vi "testSendEvtToClient.vi"(8 "error in (no error)":errorcluster) -> (0 "error out":errorcluster)   [LabVIEW 2018]
doc: "This VI generates 50 events and sends them from TCP server to TCP client."
uses:
  <vilib>/addons/_JKI Toolkits/Caraya/classes/Assert/Assert Equal Value_Variant.vi
  src/TcpServer/TcpServer.lvclass
  <vilib>/addons/_JKI Toolkits/Caraya/classes/Test/Test.lvclass
  <vilib>/addons/_JKI Toolkits/Caraya/classes/Assert/Assert.lvclass
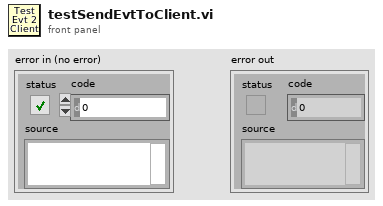
[diagram p1: front panel]
types:
  T1 = cluster{"CmdRead":refnum<user-event>, "EvtRead":refnum<user-event>, "GenRead":refnum<user-event>}
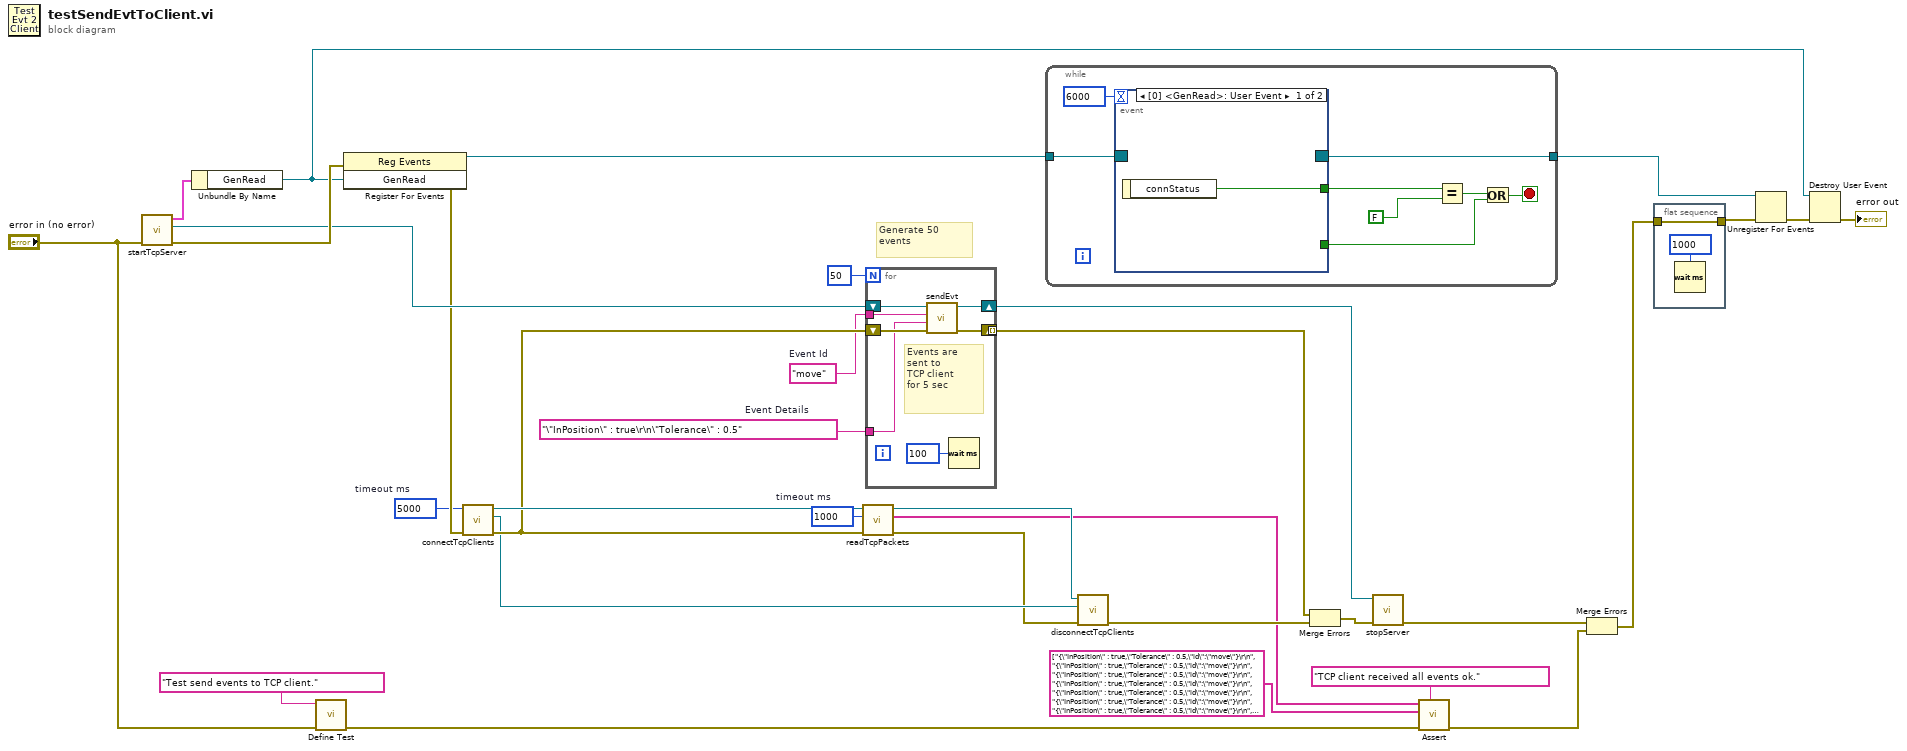
[diagram p0: block diagram]
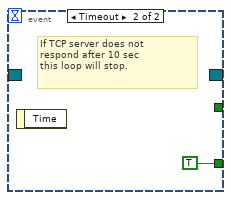
[diagram p2: hidden frame]
diagram:
  w3 = 1000  # timeout ms
  w4 = 5000  # timeout ms
  w9 = "\"InPosition\" : true\r\n\"Tolerance\" : 0.5"  # Event Details
  w8 = "move"  # Event Id
  # "Generate 50 \nevents"
  n1 = call "startTcpServer.vi"("error in (no error)"="error in (no error)") -> ("error out"=w21:errorcluster, "TcpServer out"=w18:refnum<class "TcpServer.lvclass">, "UserEvents"=w28:T1)  [unwired: 8 in]
  n2 = Unbundle By Name(w28) -> ("GenRead"=w1:refnum<user-event>)
  n3 = call <vilib>:"Define Test.vi"("error in (no error)"="error in (no error)", "Label (VI Title)"="Test send events to TCP client.") -> ("error out"=w15:errorcluster)  [unwired: 9 in]
  n4 = register-events(error in=w21, w1) -> (reference out=w33:refnum<event-registration>, error out=w10:errorcluster)  [unwired: 1 in]
  n5 = call "connectTcpClients.vi"("error in (no error)"=w10, "timeout ms"=w4) -> ("error out"=w26:errorcluster, "tel connection ID out"=w24:refnum<k5>, "cmd connection ID out"=w27:refnum<k5>)  [unwired: 7 in]
  n6 = call "readTcpPackets.vi"("error in (no error)"=w26, "timeout ms"=w3, "connection ID in"=w27) -> ("error out"=w23:errorcluster, "TCP packets"=w16:string[], "connection ID out"=w25:refnum<k5>)  [unwired: 6 in]
  n7 = for {
    N: 50 -> [_]
    tunnel: w9 -> [w35]
    tunnel: w8 -> [w40]
    shift-right: [w37] -> w11
    shift-left: w18 -> [w39]
    shift-right: [w34] -> w5
    shift-left: w26 -> [w38]
    tunnel: [w34] -> _ mode=indexing
    # "Events are\nsent to\nTCP client\nfor 5 sec"
    n8 = call "sendEvt.vi"("error in (no error)"=w38, "Event Details"=w35, "Event Id"=w40, "tcpServer in"=w39) -> ("error out"=w34:errorcluster, "tcpServer out"=w37:refnum<class "TcpServer.lvclass">)  [unwired: 6 in]
    n9 = Wait (ms)(milliseconds to wait=u32 100) -> ()  [unwired: 1 out]
  }
  n10 = while {
    tunnel: w33 -> [w48]
    tunnel: [w47] -> w32
    stop <- w42 stop-if-true
    n11 = event shown="[0] <GenRead>: User Event" {
      selector: w48 -> [_ _]
      dyn-events: [_ _] -> w47
      timeout: 6000 -> [_ _]
      tunnel: [w49 _] -> w46
      tunnel: [_ TRUE] -> w43
      event User Event {
        n12 = event-data() -> ("connStatus"=w49:bool)  [unwired: 1 in]
      }
      event Timeout {
        # "If TCP server does not\nrespond after 10 sec\nthis loop will stop."
        n13 = event-data() -> ()  [unwired: 1 in, 1 out]
      }
    }
    n14 = Equal?(x=w46, y=FALSE) -> (x = y?=w44:bool)
    n15 = Or(x=w44, y=w43) -> (x .or. y?=w42:bool)
  }
  n16 = call "disconnectTcpClients.vi"("error in (no error)"=w23, "tel connection ID in"=w24, "cmd connection ID in"=w25) -> ("error out"=w22:errorcluster)  [unwired: 8 in]
  n17 = Merge Errors(w5, w22) -> (w6:errorcluster)
  n18 = call "stopServer.vi"("error in (no error)"=w6, "tcpServer in"=w11) -> ("error out"=w30:errorcluster)  [unwired: 8 in, 1 out]
  n19 = call-poly <vilib>:"Assert.vi"("Label"="TCP client received all events ok.", "error in (no error)"=w15, "Y"=string[] ["{\"InPosition\" : true,\"Tolerance\" : 0.5,\"id\":\"move\"}\r\n", "{\"InPosition\" : true,\"Tolerance\" : 0.5,\"id\":\"move\"}\r\n", "{\"InPosition\" : true,\"Tolerance\" : 0.5,\"id\":\"move\"}\r\n", "{\"InPosition\" : true,\"Tolerance\" : 0.5,\"id\":\"move\"}\r\n", "{\"InPosition\" : true,\"Tolerance\" : 0.5,\"id\":\"move\"}\r\n", "{\"InPosition\" : true,\"Tolerance\" : 0.5,\"id\":\"move\"}\r\n", "{\"InPosition\" : true,\"Tolerance\" : 0.5,\"id\":\"move\"}\r\n", "{\"InPosition\" : true,\"Tolerance\" : 0.5,\"id\":\"move\"}\r\n", "{\"InPosition\" : true,\"Tolerance\" : 0.5,\"id\":\"move\"}\r\n", "{\"InPosition\" : true,\"Tolerance\" : 0.5,\"id\":\"move\"}\r\n", "{\"InPosition\" : true,\"Tolerance\" : 0.5,\"id\":\"move\"}\r\n", "{\"InPosition\" : true,\"Tolerance\" : 0.5,\"id\":\"move\"}\r\n", "{\"InPosition\" : true,\"Tolerance\" : 0.5,\"id\":\"move\"}\r\n", "{\"InPosition\" : true,\"Tolerance\" : 0.5,\"id\":\"move\"}\r\n", "{\"InPosition\" : true,\"Tolerance\" : 0.5,\"id\":\"move\"}\r\n", "{\"InPosition\" : true,\"Tolerance\" : 0.5,\"id\":\"move\"}\r\n", "{\"InPosition\" : true,\"Tolerance\" : 0.5,\"id\":\"move\"}\r\n", "{\"InPosition\" : true,\"Tolerance\" : 0.5,\"id\":\"move\"}\r\n", "{\"InPosition\" : true,\"Tolerance\" : 0.5,\"id\":\"move\"}\r\n", "{\"InPosition\" : true,\"Tolerance\" : 0.5,\"id\":\"move\"}\r\n", "{\"InPosition\" : true,\"Tolerance\" : 0.5,\"id\":\"move\"}\r\n", "{\"InPosition\" : true,\"Tolerance\" : 0.5,\"id\":\"move\"}\r\n", "{\"InPosition\" : true,\"Tolerance\" : 0.5,\"id\":\"move\"}\r\n", "{\"InPosition\" : true,\"Tolerance\" : 0.5,\"id\":\"move\"}\r\n", "{\"InPosition\" : true,\"Tolerance\" : 0.5,\"id\":\"move\"}\r\n", "{\"InPosition\" : true,\"Tolerance\" : 0.5,\"id\":\"move\"}\r\n", "{\"InPosition\" : true,\"Tolerance\" : 0.5,\"id\":\"move\"}\r\n", "{\"InPosition\" : true,\"Tolerance\" : 0.5,\"id\":\"move\"}\r\n", "{\"InPosition\" : true,\"Tolerance\" : 0.5,\"id\":\"move\"}\r\n", "{\"InPosition\" : true,\"Tolerance\" : 0.5,\"id\":\"move\"}\r\n", "{\"InPosition\" : true,\"Tolerance\" : 0.5,\"id\":\"move\"}\r\n", "{\"InPosition\" : true,\"Tolerance\" : 0.5,\"id\":\"move\"}\r\n", "{\"InPosition\" : true,\"Tolerance\" : 0.5,\"id\":\"move\"}\r\n", "{\"InPosition\" : true,\"Tolerance\" : 0.5,\"id\":\"move\"}\r\n", "{\"InPosition\" : true,\"Tolerance\" : 0.5,\"id\":\"move\"}\r\n", "{\"InPosition\" : true,\"Tolerance\" : 0.5,\"id\":\"move\"}\r\n", "{\"InPosition\" : true,\"Tolerance\" : 0.5,\"id\":\"move\"}\r\n", "{\"InPosition\" : true,\"Tolerance\" : 0.5,\"id\":\"move\"}\r\n", "{\"InPosition\" : true,\"Tolerance\" : 0.5,\"id\":\"move\"}\r\n", "{\"InPosition\" : true,\"Tolerance\" : 0.5,\"id\":\"move\"}\r\n", "{\"InPosition\" : true,\"Tolerance\" : 0.5,\"id\":\"move\"}\r\n", "{\"InPosition\" : true,\"Tolerance\" : 0.5,\"id\":\"move\"}\r\n", "{\"InPosition\" : true,\"Tolerance\" : 0.5,\"id\":\"move\"}\r\n", "{\"InPosition\" : true,\"Tolerance\" : 0.5,\"id\":\"move\"}\r\n", "{\"InPosition\" : true,\"Tolerance\" : 0.5,\"id\":\"move\"}\r\n", "{\"InPosition\" : true,\"Tolerance\" : 0.5,\"id\":\"move\"}\r\n", "{\"InPosition\" : true,\"Tolerance\" : 0.5,\"id\":\"move\"}\r\n", "{\"InPosition\" : true,\"Tolerance\" : 0.5,\"id\":\"move\"}\r\n", "{\"InPosition\" : true,\"Tolerance\" : 0.5,\"id\":\"move\"}\r\n", "{\"InPosition\" : true,\"Tolerance\" : 0.5,\"id\":\"move\"}\r\n"] ("array w/ subset deleted"), "X"=w16) -> ("error out"=w13:errorcluster)  [unwired: 7 in]
  n20 = Merge Errors(w30, w13) -> (w14:errorcluster)
  n21 = flat-sequence {
    tunnel: w14 -> [w51]
    tunnel: [w51] -> w29
    frame #0 {
      n22 = Wait (ms)(milliseconds to wait=u32 1000) -> ()  [unwired: 1 out]
    }
  }
  n23 = Unregister For Events(event registration refnum=w32, error in=w29) -> (error out=w31:errorcluster)
  n24 = Destroy User Event(user event=w1, error in=w31) -> (error out=→"error out":errorcluster)
